vi "New Server from Socket.vi"(8 "error in (no error)":errorcluster, 11 "Socket":refnum<class "Socket.lvclass">) -> (0 "error out":errorcluster, 3 "WebSocket Server out":refnum<class "WebSocket Server.lvclass">)   [LabVIEW 2013, in "WebSockets.lvlib" / "WebSocket Server.lvclass"]
doc: "Creates a new WebSocket Server connection from an existing Socket connection."
uses:
  WebSocket Server.lvclass
  Sockets/Socket/Socket.lvclass
  WebSocket/WebSocket.lvclass/WebSocket.ctl
  WebSocket/Write Socket.vi
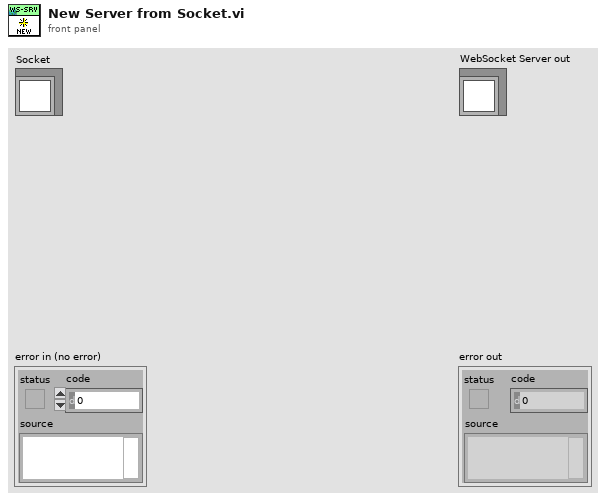
[diagram p1: front panel]
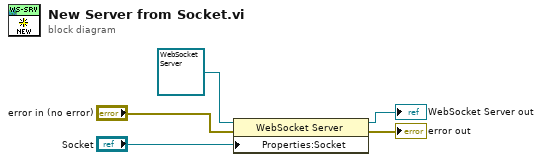
[diagram p0: block diagram]
diagram:
  n1 = property class="WebSocket Server"(reference=refnum<class "WebSocket Server.lvclass"> refnum ("WebSocket Server out"), error in="error in (no error)", "Properties:Socket"="Socket") -> (reference out=→"WebSocket Server out":refnum<class "WebSocket Server.lvclass">, error out=→"error out":errorcluster)
